vi "Basic Test 3.vi"() -> ()   [LabVIEW 2014, in "ESP8266 WiFi Wrapper.lvlib"]
uses:
  ESP8266 WiFi Wrapper.lvlib
panel:
  in  "Listen Port":u8=80
  in  "WiFi Server Mode":T1(ring)=enum."WIFI_AP"
  in  "Password":string="secretcave"
  in  "SSID":string="SecretCave with Apples"
  out "Error Out":errorcluster
  in  "Error In":errorcluster
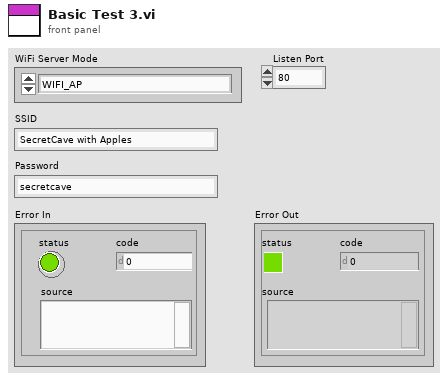
[diagram p1: front panel]
types:
  T1 = enum16{"WIFI_OFF", "WIFI_STA", "WIFI_AP", "WIFI_AP_STA"}
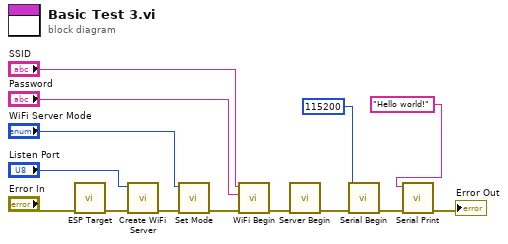
[diagram p0: block diagram]
diagram:
  n1 = call "ESP Target.vi"("Error In"="Error In") -> ("Error Out"=w2:errorcluster)  [unwired: 10 in]
  n2 = call "Create WiFi Server.vi"("Error In"=w2, "Listen Port"="Listen Port") -> ("Error Out"=w14:errorcluster)  [unwired: 9 in]
  n3 = call "Set Mode.vi"("Error In"=w14, "WiFi Server Mode"="WiFi Server Mode") -> ("Error Out"=w13:errorcluster)  [unwired: 9 in]
  n4 = call "WiFi Begin.vi"("Error In"=w13, "Password"="Password", "SSID"="SSID") -> ("Error Out"=w8:errorcluster)  [unwired: 8 in]
  n5 = call "Server Begin.vi"("Error In"=w8) -> ("Error Out"=w7:errorcluster)  [unwired: 10 in]
  n6 = call "Serial Begin.vi"("Error In"=w7, "Speed"=u32 115200) -> ("Error Out"=w6:errorcluster)  [unwired: 9 in]
  n7 = call "Serial Print.vi"("Error In"=w6, "String to print"="Hello world!") -> ("Error Out"=→"Error Out":errorcluster)  [unwired: 9 in]
